vi "Both Beam Breaker test.vi"() -> ()   [LabVIEW 2014]
panel:
  out "Arm Beam Breaker":bool
  out "Tote Beam Breaker":bool
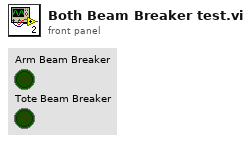
[diagram p1: front panel]
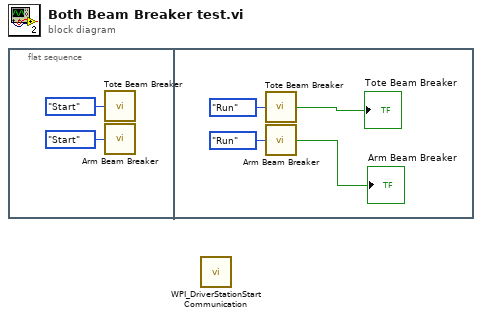
[diagram p0: block diagram]
diagram:
  n1 = flat-sequence {
    frame #0 {
      n2 = call "Tote Beam Breaker.vi"("Mode"=enum8{"Start", "Run", "Finish"}."Start") -> ()  [unwired: 1 out]
      n3 = call "Arm Beam Breaker.vi"("Mode"=enum8{"Start", "Run", "Finish"}."Start") -> ()  [unwired: 1 out]
    }
    frame #1 {
      n4 = call "Tote Beam Breaker.vi"("Mode"=enum8{"Start", "Run", "Finish"}."Run") -> ("Tote Beam Breaker"=→"Tote Beam Breaker":bool)
      n5 = call "Arm Beam Breaker.vi"("Mode"=enum8{"Start", "Run", "Finish"}."Run") -> ("Arm Beam Breaker"=→"Arm Beam Breaker":bool)
    }
  }
  n6 = call <vilib>:"WPI_DriverStationStart Communication.vi"() -> ()  [unwired: 12 in]
